vi "email data error.vi"(9 "Data Status":T3, 10 "data server":string="128.84.245.227", 11 "Process Method":T1={"Operator information"=[], "data log interval"=5, "data loop interval"=20, "Datalog directory path"=path "", "graph update interval"=1.0, "history length"=1000, "Control Logic file path"=path "C:/Documents and Settings/mw24/Desktop/rules.rul", "Sensor Configuration file path"=path "", "HMI VI path"=path "", "HMI data smooth"=0.1} {"HMI data smooth" min=0.01 format="%.2f"; "history length" min=1; "graph update interval" min=0.1 format="%.2f"; "data log interval" min=1}) -> ()   [LabVIEW 2010]
uses:
  data status.ctl
  Plant method.ctl
  operator info.ctl
  <vilib>/Utility/SMTP/NI_SMTPEmail.lvlib
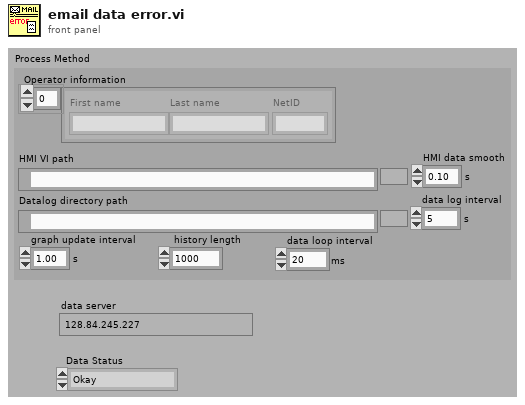
[diagram p1: front panel]
types:
  T1 = typedef "Plant method.ctl" = cluster{"Operator information":T2, "data log interval":u32, "data loop interval":u32, "Datalog directory path":path, "graph update interval":sgl, "history length":u16, "Control Logic file path":path, "Sensor Configuration file path":path, "HMI VI path":path, "HMI data smooth":dbl}
  T2 = typedef "operator info.ctl" = cluster{"First name":string, "Last name":string, "NetID":string}[]
  T3 = typedef "data status.ctl" = enum16{"Okay", "Sensor Range error", "Server error"}
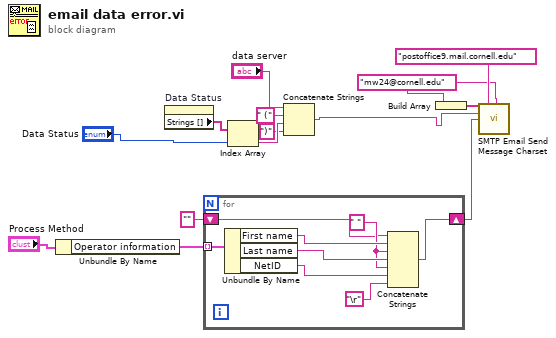
[diagram p0: block diagram]
diagram:
  w12 = "mw24@cornell.edu"
  n1 = Unbundle By Name("Process Method") -> ("Operator information"=w4:T2)
  n2 = property on="Data Status" class="Enum (strict)"() -> ("Strings []"=w11:string[])  [unwired: 2 in, 2 out]
  n3 = for {
    tunnel: w4 -> [w22] mode=indexing
    shift-right: [w16] -> w2
    shift-left: "" -> [w15]
    w18 = " " ("string")
    n4 = Unbundle By Name(w22) -> ("First name"=w21:string, "Last name"=w20:string, "NetID"=w19:string)
    n5 = Concatenate Strings(w15, w21, w18, w20, w18, w19, "\r") -> (w16:string)
  }
  n6 = Index Array(array=w11, index="Data Status") -> (element=w7:string)
  n7 = Concatenate Strings("data server", " (" ("string"), w7, ")" ("string")) -> (w5:string)
  n8 = Build Array(w12) -> (w13:string[])
  n9 = call <vilib>:"SMTP Email Send Message Charset.vi"("recipients"=w13, "mail server"="postoffice9.mail.cornell.edu", "return address"=w12, "subject ([No Subject])"=w5, "message"=w2) -> ()  [unwired: 9 in, 2 out]
